vi "Dialog_ImageNotUptodate_Error.vi"() -> ()   [LabVIEW 2012]
panel:
  in  "OK Button":bool
  # "'Current Image' not up-to-date!"
  # "Focus at current position first."
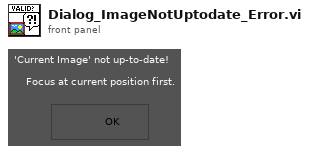
[diagram p1: front panel]
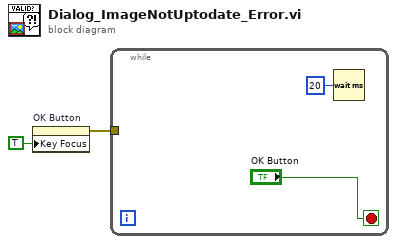
[diagram p0: block diagram]
diagram:
  n1 = property on="OK Button" class="Bool"("Key Focus"=TRUE) -> (error out=w1:errorcluster)  [unwired: 2 in, 1 out]
  n2 = while {
    tunnel: w1 -> [_]
    stop <- "OK Button" stop-if-true
    n3 = Wait (ms)(milliseconds to wait=u32 20) -> ()  [unwired: 1 out]
  }
